vi "Updater Remove Client INI File.vi"(8 "error in (no error)":errorcluster, 11 "Spartan Install Path":path) -> (0 "error out":errorcluster)   [LabVIEW 2011]
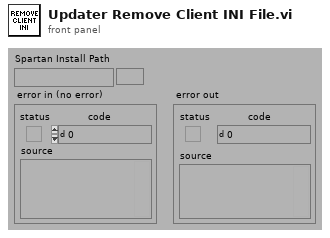
[diagram p1: front panel]
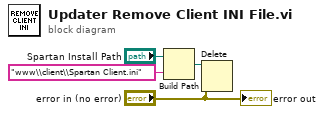
[diagram p0: block diagram]
diagram:
  n1 = Build Path(base path="Spartan Install Path", name or relative path="www\\client\\Spartan Client.ini") -> (appended path=w2:path)
  n2 = Delete(path (use dialog)=w2, error in="error in (no error)") -> ()  [unwired: 6 out]
  "error out" <- "error in (no error)"
